vi "6 motor auton thing.vi"(0 "Left Motor 1":string, 1 "Left Motor 2":string, 2 "Left Motor 3":string, 3 "Right Motor 1":string, 4 "Right Motor 2":string, 5 "Right Motor 3":string, 6 "Encoder 1":string, 7 "Encoder 4":string, 8 "Encoder 2":string, 9 "Encoder 5":string, 10 "Encoder 3":string, 11 "Encoder 6":string, 12 "Speed":dbl, 13 "Distance":dbl) -> ()   [LabVIEW 2017]
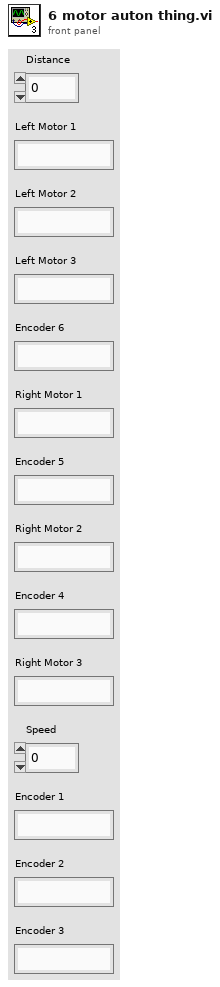
[diagram p1: front panel]
types:
  T1 = typedef "WPI_EncoderDevRef.ctl" = cluster{"DevStatus":errorcluster, "EncoderIndex":T2, "CounterIndex":T3, "DistancePerCount":dbl, "Decoding Type":T4}
  T2 = typedef "FPGA_EncoderIdx.ctl" = enum8{"Enc 0", "Enc 1", "Enc 2", "Enc 3", "Enc 4", "Enc 5", "Enc 6", "Enc 7", "Invalid"}
  T3 = typedef "FPGA_CounterCtrSystemIndex.ctl" = enum8{"Ctr 0", "Ctr 1", "Ctr 2", "Ctr 3", "Ctr 4", "Ctr 5", "Ctr 6", "Ctr 7", "Invalid"}
  T4 = typedef "WPI_EncoderType.ctl" = enum16{"1x", "2x", "4x"}
  T5 = typedef "WPI_MotorControlDeviceRef.ctl" = cluster{"DeviceStatus":errorcluster, "Type":T6, "PWM":cluster{"PWM Channel":T7, "DeadBand":T8}, "CAN":cluster{"Device Number":u8, "SetOutput VI Ref":variant, "GetOutput VI Ref":variant, "Enable VI Ref":variant, "Disable VI Ref":variant, "Data":variant}, "Invert":bool, "DIO PWM":cluster{"PWM \"Enable\" Channel":T7, "DIOChannel":T9, "PWM Rate":dbl}}
  T6 = typedef "WPI_MotorControlType.ctl" = enum16{"PWM", "CAN", "DIO PWM"}
  T7 = typedef "FPGA_DIOPWMChannel.ctl" = enum8{"PWM 0", "PWM 1", "PWM 2", "PWM 3", "PWM 4", "PWM 5", "PWM 6", "PWM 7", "PWM 8", "PWM 9", "PWM MXP 0", "PWM MXP 1", "PWM MXP 2", "PWM MXP 3", "PWM MXP 4", "PWM MXP 5", "PWM MXP 6", "PWM MXP 7", "PWM MXP 8", "PWM MXP 9", "Invalid"}
  T8 = typedef "WPI_PWMDeadband.ctl" = cluster{"Name":string, "maxPositivePwm":i32, "minPositivePwm":i32, "centerPwm":i32, "maxNegativePwm":i32, "minNegativePwm":i32, "angularRange":u16}
  T9 = typedef "FPGA_DIOChannel.ctl" = enum8{"DIO 0", "DIO 1", "DIO 2", "DIO 3", "DIO 4", "DIO 5", "DIO 6", "DIO 7", "DIO 8", "DIO 9", "DIO MXP 0", "DIO MXP 1", "DIO MXP 2", "DIO MXP 3", "DIO MXP 4", "DIO MXP 5", "DIO MXP 6", "DIO MXP 7", "DIO MXP 8", "DIO MXP 9", "DIO MXP 10", "DIO MXP 11", "DIO MXP 12", "DIO MXP 13", "DIO MXP 14", "DIO MXP 15", "SPI Port CS1", "SPI Port CS2", "SPI Port CS3", "SPI Port MISO", "SPI Port MOSI", "Invalid"}
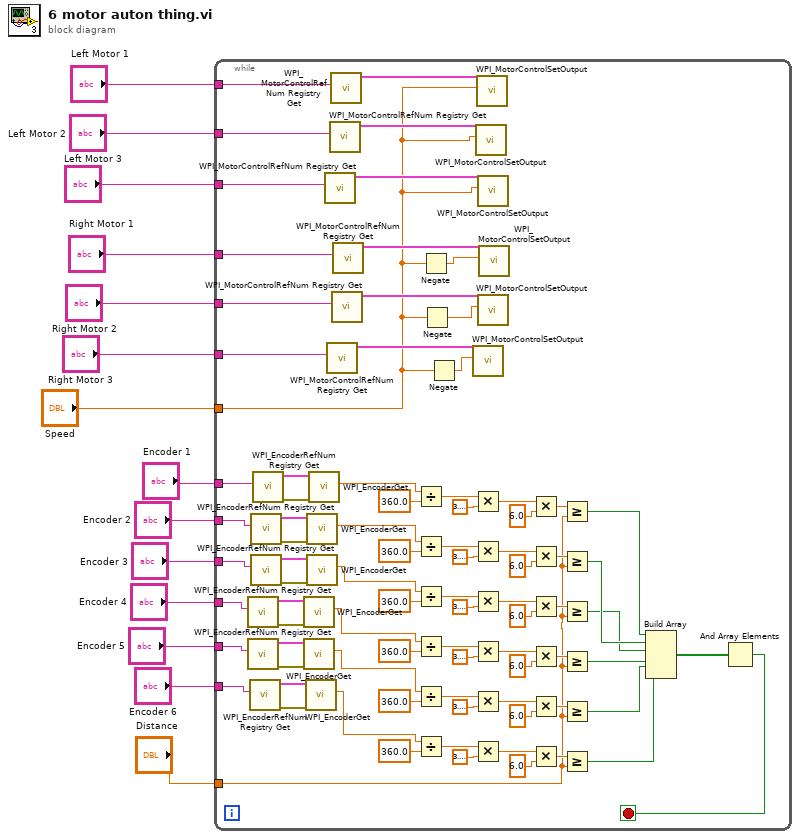
[diagram p0: block diagram]
diagram:
  n1 = while {
    tunnel: "Left Motor 3" -> [w99]
    tunnel: "Left Motor 2" -> [w96]
    tunnel: "Right Motor 1" -> [w93]
    tunnel: "Right Motor 2" -> [w92]
    tunnel: "Right Motor 3" -> [w89]
    tunnel: "Left Motor 1" -> [w88]
    tunnel: "Speed" -> [w40]
    tunnel: "Encoder 1" -> [w27]
    tunnel: "Encoder 2" -> [w26]
    tunnel: "Encoder 3" -> [w25]
    tunnel: "Encoder 4" -> [w24]
    tunnel: "Encoder 5" -> [w23]
    tunnel: "Encoder 6" -> [w22]
    tunnel: "Distance" -> [w15]
    stop <- w44 stop-if-true
    n2 = call <vilib>:"WPI_EncoderRefNum Registry Get.vi"("refnum name"=w24) -> ("error out"=w35:errorcluster, "EncoderDevRef"=w34:T1)  [unwired: 9 in]
    n3 = call <vilib>:"WPI_EncoderRefNum Registry Get.vi"("refnum name"=w23) -> ("error out"=w36:errorcluster, "EncoderDevRef"=w37:T1)  [unwired: 9 in]
    n4 = call <vilib>:"WPI_EncoderRefNum Registry Get.vi"("refnum name"=w22) -> ("error out"=w39:errorcluster, "EncoderDevRef"=w38:T1)  [unwired: 9 in]
    n5 = call <vilib>:"WPI_EncoderRefNum Registry Get.vi"("refnum name"=w26) -> ("error out"=w31:errorcluster, "EncoderDevRef"=w30:T1)  [unwired: 9 in]
    n6 = call <vilib>:"WPI_EncoderRefNum Registry Get.vi"("refnum name"=w25) -> ("error out"=w32:errorcluster, "EncoderDevRef"=w33:T1)  [unwired: 9 in]
    n7 = call <vilib>:"WPI_EncoderRefNum Registry Get.vi"("refnum name"=w27) -> ("error out"=w28:errorcluster, "EncoderDevRef"=w29:T1)  [unwired: 9 in]
    n8 = call <vilib>:"WPI_EncoderGet.vi"("error in (no error)"=w35, "EncoderDevRef"=w34) -> ("Distance"=w18:dbl)  [unwired: 4 in, 5 out]
    n9 = call <vilib>:"WPI_EncoderGet.vi"("error in (no error)"=w36, "EncoderDevRef"=w37) -> ("Distance"=w17:dbl)  [unwired: 4 in, 5 out]
    n10 = call <vilib>:"WPI_EncoderGet.vi"("error in (no error)"=w39, "EncoderDevRef"=w38) -> ("Distance"=w16:dbl)  [unwired: 4 in, 5 out]
    n11 = call <vilib>:"WPI_EncoderGet.vi"("error in (no error)"=w31, "EncoderDevRef"=w30) -> ("Distance"=w20:dbl)  [unwired: 4 in, 5 out]
    n12 = call <vilib>:"WPI_EncoderGet.vi"("error in (no error)"=w32, "EncoderDevRef"=w33) -> ("Distance"=w19:dbl)  [unwired: 4 in, 5 out]
    n13 = call <vilib>:"WPI_EncoderGet.vi"("error in (no error)"=w28, "EncoderDevRef"=w29) -> ("Distance"=w21:dbl)  [unwired: 4 in, 5 out]
    n14 = call <vilib>:"WPI_MotorControlRefNum Registry Get.vi"("refnum name"=w99) -> ("MotorControlDevRef"=w98:T5)  [unwired: 9 in, 1 out]
    n15 = call <vilib>:"WPI_MotorControlRefNum Registry Get.vi"("refnum name"=w89) -> ("MotorControlDevRef"=w90:T5)  [unwired: 9 in, 1 out]
    n16 = call <vilib>:"WPI_MotorControlRefNum Registry Get.vi"("refnum name"=w96) -> ("MotorControlDevRef"=w97:T5)  [unwired: 9 in, 1 out]
    n17 = call <vilib>:"WPI_MotorControlRefNum Registry Get.vi"("refnum name"=w88) -> ("MotorControlDevRef"=w95:T5)  [unwired: 9 in, 1 out]
    n18 = call <vilib>:"WPI_MotorControlRefNum Registry Get.vi"("refnum name"=w92) -> ("MotorControlDevRef"=w91:T5)  [unwired: 9 in, 1 out]
    n19 = call <vilib>:"WPI_MotorControlRefNum Registry Get.vi"("refnum name"=w93) -> ("MotorControlDevRef"=w94:T5)  [unwired: 9 in, 1 out]
    n20 = Divide(x=w21, y=360.0) -> (x/y=w85:dbl)
    n21 = Divide(x=w20, y=360.0) -> (x/y=w80:dbl)
    n22 = Divide(x=w19, y=360.0) -> (x/y=w75:dbl)
    n23 = Divide(x=w18, y=360.0) -> (x/y=w70:dbl)
    n24 = Divide(x=w17, y=360.0) -> (x/y=w65:dbl)
    n25 = Divide(x=w16, y=360.0) -> (x/y=w60:dbl)
    n26 = Negate(x=w40) -> (-x=w43:dbl)
    n27 = Negate(x=w40) -> (-x=w41:dbl)
    n28 = Negate(x=w40) -> (-x=w42:dbl)
    n29 = call <vilib>:"WPI_MotorControlSetOutput.vi"("Output"=w42, "MotorControlDevRef"=w90) -> ()  [unwired: 7 in, 3 out]
    n30 = Multiply(x=w85, y=3.141592653589793) -> (x*y=w84:dbl)
    n31 = Multiply(x=w80, y=3.141592653589793) -> (x*y=w81:dbl)
    n32 = Multiply(x=w75, y=3.141592653589793) -> (x*y=w74:dbl)
    n33 = Multiply(x=w70, y=3.141592653589793) -> (x*y=w71:dbl)
    n34 = Multiply(x=w65, y=3.141592653589793) -> (x*y=w64:dbl)
    n35 = Multiply(x=w60, y=3.141592653589793) -> (x*y=w61:dbl)
    n36 = call <vilib>:"WPI_MotorControlSetOutput.vi"("Output"=w40, "MotorControlDevRef"=w97) -> ()  [unwired: 7 in, 3 out]
    n37 = call <vilib>:"WPI_MotorControlSetOutput.vi"("Output"=w40, "MotorControlDevRef"=w95) -> ()  [unwired: 7 in, 3 out]
    n38 = call <vilib>:"WPI_MotorControlSetOutput.vi"("Output"=w40, "MotorControlDevRef"=w98) -> ()  [unwired: 7 in, 3 out]
    n39 = call <vilib>:"WPI_MotorControlSetOutput.vi"("Output"=w41, "MotorControlDevRef"=w91) -> ()  [unwired: 7 in, 3 out]
    n40 = call <vilib>:"WPI_MotorControlSetOutput.vi"("Output"=w43, "MotorControlDevRef"=w94) -> ()  [unwired: 7 in, 3 out]
    n41 = Multiply(x=w84, y=6.0) -> (x*y=w57:dbl)
    n42 = Multiply(x=w81, y=6.0) -> (x*y=w56:dbl)
    n43 = Multiply(x=w74, y=6.0) -> (x*y=w55:dbl)
    n44 = Multiply(x=w71, y=6.0) -> (x*y=w54:dbl)
    n45 = Multiply(x=w64, y=6.0) -> (x*y=w53:dbl)
    n46 = Multiply(x=w61, y=6.0) -> (x*y=w52:dbl)
    n47 = Greater Or Equal?(x=w57, y=w15) -> (x >= y?=w51:bool)
    n48 = Greater Or Equal?(x=w56, y=w15) -> (x >= y?=w50:bool)
    n49 = Greater Or Equal?(x=w55, y=w15) -> (x >= y?=w49:bool)
    n50 = Greater Or Equal?(x=w54, y=w15) -> (x >= y?=w48:bool)
    n51 = Greater Or Equal?(x=w53, y=w15) -> (x >= y?=w47:bool)
    n52 = Greater Or Equal?(x=w52, y=w15) -> (x >= y?=w46:bool)
    n53 = Build Array(w51, w50, w49, w48, w47, w46) -> (w45:bool[])
    n54 = And Array Elements(Boolean array=w45) -> (logical AND=w44:bool)
  }
